vi "Process File.vi"(8 "error in (no error)":errorcluster, 10 "Result in":refnum<class "Acquired Result.lvclass">, 11 "Log Record in":refnum<class "Log Record.lvclass">) -> (0 "error out":errorcluster, 2 "Result out":refnum<class "Acquired Result.lvclass">, 3 "Log Record out":refnum<class "Log Record.lvclass">)   [LabVIEW 2024, in "Log Record.lvclass"]
uses:
  Log Record.lvclass
  NHMFL_Core/Libraries/Instruments/Results/Acquired Result/Acquired Result.lvclass
  Log Record.lvclass/Log Record.ctl
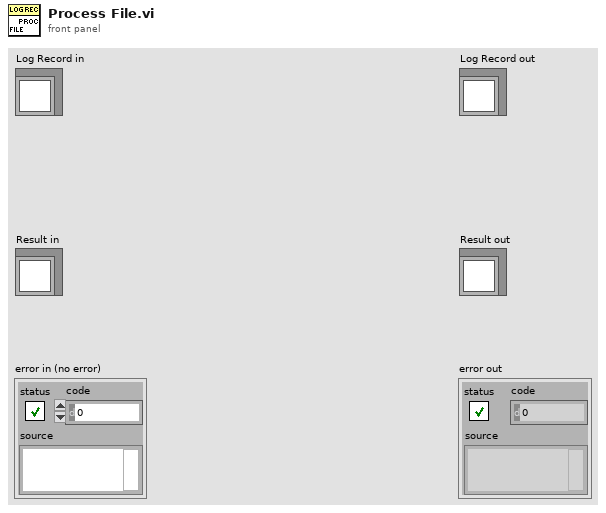
[diagram p1: front panel]
types:
  T1 = typedef "Log Record State.ctl" = enum16{"Idle", "Requested login", "Logged on", "Requested logout", "Logged off"}
  T2 = typedef "Add-on Storage.ctl" = enum16{"OSF", "OSF - Split", "Google Drive", "Dropbox", "Box"}
  T3 = typedef "Log Record Configuration.ctl" = cluster{"OSF node  ID":string, "Conection timeout":dbl, "Station":string, "Log server ":string, "Upload to OSF":bool, "Append to lab book":bool, "Filing modules":string[], "File prefix":string, "Computer":string}
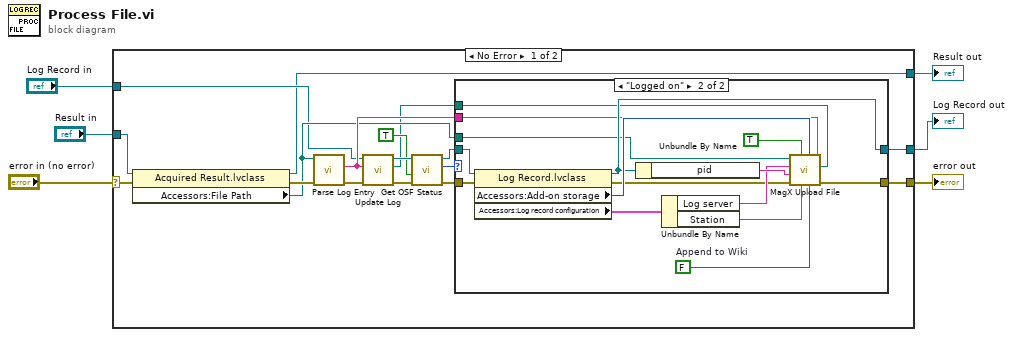
[diagram p0: block diagram]
diagram:
  n1 = case shown="No Error" "error in (no error)" {
    selector: "error in (no error)" -> [w18 w43]
    tunnel: "Result in" -> [w10 w41]
    tunnel: [w23 w43] -> w5
    tunnel: [w9 w41] -> w4
    tunnel: [w22 w42] -> w3
    tunnel: "Log Record in" -> [w11 w42]
    frame No Error {
      n2 = property class="Acquired Result.lvclass"(reference=w10, error in=w18) -> (reference out=w9:refnum<class "Acquired Result.lvclass">, error out=w17:errorcluster, "Accessors:File Path"=w12:path)
      n3 = call "Parse Log Entry.vi"("error in"=w17, "File name"=w12) -> ("error out"=w16:errorcluster, "Lab notebook entry"=w13:string)  [unwired: 8 in]
      n4 = call-dynamic "Update Log.vi"("error in (no error)"=w16, "Lab notebook entry"=w13, "Log Record in"=w11) -> ("error out"=w14:errorcluster, "path"=w7:path, "Log Record out"=w15:refnum<class "Log Record.lvclass">)  [unwired: 6 in]
      n5 = call-dynamic "Get OSF Status.vi"("error in (no error)"=w14, "Skip if offline"=TRUE, "Log Record in"=w15) -> ("error out"=w20:errorcluster, "State"=w19:T1, "Log Record out"=w21:refnum<class "Log Record.lvclass">)  [unwired: 6 in]
      n6 = case shown="\"Logged on\"" w19 {
        tunnel: [w25 w31] -> w23
        tunnel: [w24 w32] -> w22
        tunnel: w21 -> [w24 w36]
        tunnel: w20 -> [w25 w35]
        tunnel: w13 -> [_ w29]
        tunnel: w12 -> [_ w28]
        tunnel: w7 -> [_ w27]
        frame "Idle", Default {
        }
        frame "Logged on" {
          w26 = FALSE  # Append to Wiki
          n7 = property class="Log Record.lvclass"(reference=w36, error in=w35) -> (reference out=w32:refnum<class "Log Record.lvclass">, error out=w30:errorcluster, "Accessors:Add-on storage"=w33:T2, "Accessors:Log record configuration"=w34:T3)
          n8 = Unbundle By Name(w32) -> ("pid"=w40:string)
          n9 = Unbundle By Name(w34) -> ("Log server"=w39:string, "Station"=w38:string)
          n10 = call "MagX Upload File.vi"("Log File"=w27, "Lab notebook entry"=w29, "Append to Wiki"=w26, "Add-on storage"=w33, "Station"=w38, "Create Markdown"=TRUE ("Append to Wiki"), "error in"=w30, "Experiment ID"=w40, "Log server"=w39, "File name"=w28) -> ("error out"=w31:errorcluster)  [unwired: 1 in]
        }
      }
    }
    frame Error {
    }
  }
  "error out" <- w5
  "Log Record out" <- w3
  "Result out" <- w4
